vi "Calibration-Frame15.vi"(8 "Reset Measurement Prog":bool, 9 "Array 8":dbl[](array[numeric]), 10 "data mode":enum16{"Take new data point", "Refit Curve"}(ring), 11 "Results file output":path) -> ()   [LabVIEW 2022 SP3]
uses:
  Anemometry Sub Vis/Globals/Calib_global.vi
  Anemometry Sub Vis/Controls/App_Global.ctl
  Anemometry Sub Vis/Controls/Setup.ctl
  Anemometry Sub Vis/Controls/Post_Process.ctl
  Anemometry Sub Vis/Controls/Save_Data.ctl
  Anemometry Sub Vis/File/Setup_Filetype.ctl
  Anemometry Sub Vis/Globals/Meas_global.vi
  Anemometry Sub Vis/Controls/Inst_type.ctl
  Anemometry Sub Vis/Controls/portOrDev.ctl
  Anemometry Sub Vis/Controls/calType.ctl
  Anemometry Sub Vis/Controls/channelState.ctl
  Anemometry Sub Vis/Controls/Meas input Cluster.ctl
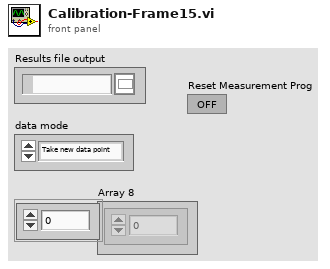
[diagram p1: front panel]
types:
  T1 = typedef "App_Global.ctl" = enum16{"Read Global", "Write to Global", "Initialise Array"}
  T2 = typedef "Save_Data.ctl" = enum16{"Save No Data", "Save Data"}
  T3 = typedef "Post_Process.ctl" = enum16{"Take New Data", "Post Process Raw Data File"}
  T4 = typedef "Setup.ctl" = enum16{"Run Program", "Show Setup", "Save Current Setup", "Setup Front Panel"}
  T5 = typedef "Setup_Filetype.ctl" = enum16{"Measurement Setups", "Calibration Setups", "General", "Results File Plotter Setups", "Speed Calib Tweaks"}
  T6 = typedef "Meas input Cluster.ctl" = cluster{"Type":T7, "Label":string, "DAQ":string, "Port":T8, "Ch":i32, "Cal":path, "calType":T9, "Fs":dbl, "syncDelay":dbl, "chState":T10}
  T7 = typedef "Inst_type.ctl" = enum16{"Raw voltage", "Raw with zero offsetting", "Propeller anemometer", "Pressure Transducer", "Pitot-static tube", "Hot wire", "Cross wire 1", "Cross wire 2", "Generic Linear", "Generic Polynomial", "Generic BackPoly", "Fast FID", "Thermocouple", "Cold wire", "Pulsed Wire", "LDA Vel", "LDA Tran time", "LDA Arr time", "Microphone"}
  T8 = typedef "portOrDev.ctl" = string
  T9 = typedef "calType.ctl" = enum32{"Latest", "Fixed"}
  T10 = typedef "channelState.ctl" = enum32{"No Selection", "Solo", "Mute"}
  T11 = typedef "Cal_Inst_type.ctl" = enum16{"Propeller anemometer", "Pressure Transducer", "Hot wire", "Cross wire velocity", "Cross wire angle", "Generic Linear", "Generic Polynomial", "Poly Fit Special", "Fast FID", "Thermocouple", "Cold wire", "Pulsed Wire"}
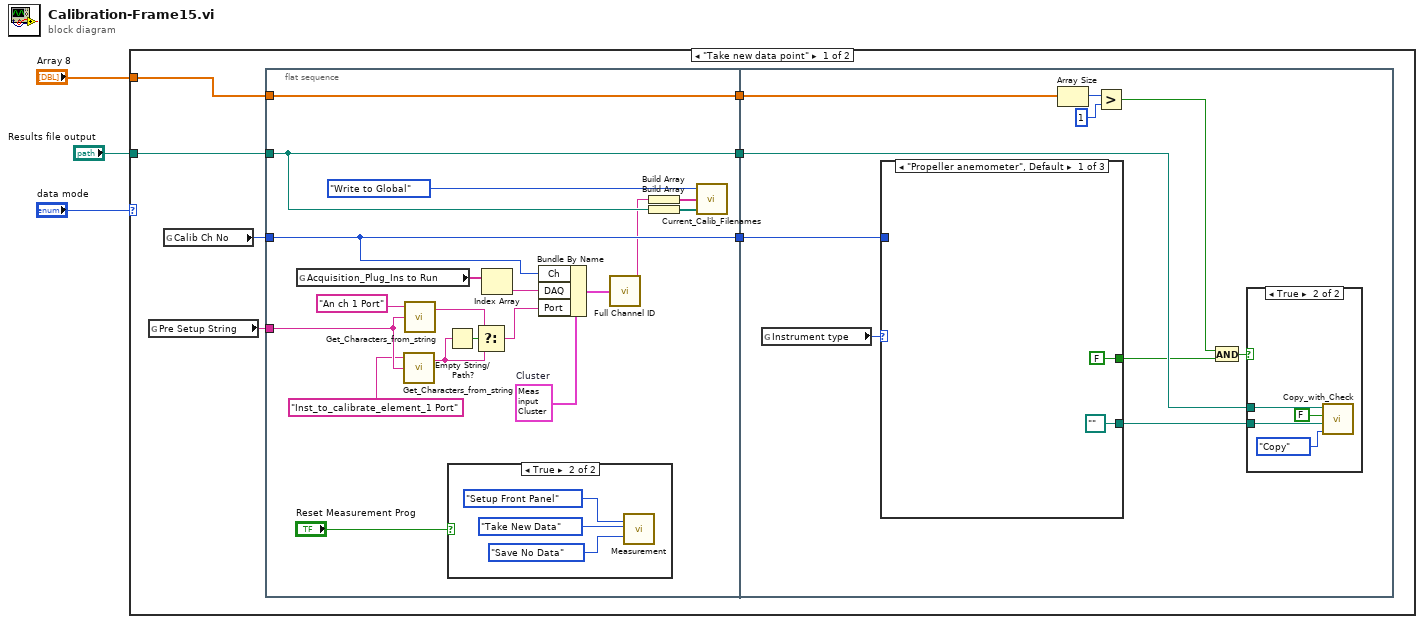
[diagram p0: block diagram]
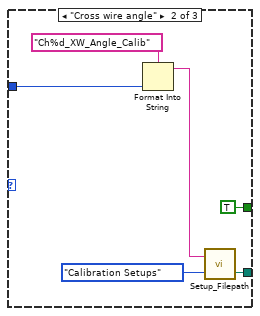
[diagram p4: hidden frame]
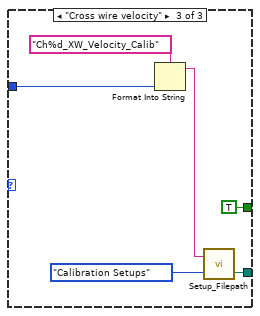
[diagram p5: hidden frame]
diagram:
  n1 = case shown="\"Take new data point\"" "data mode" {
    tunnel: "Results file output" -> [w10 _]
    tunnel: "Array 8" -> [w6 _]
    frame "Take new data point" {
      n2 = global read "Calib_global.vi" "Pre Setup String"() -> (w4:string)
      n3 = global read "Calib_global.vi" "Calib Ch No"() -> (w9:i16)
      n4 = flat-sequence {
        tunnel: w10 -> [w26]
        tunnel: [w26] -> w8
        tunnel: w9 -> [w20]
        tunnel: [w20] -> w7
        tunnel: w6 -> [w25]
        tunnel: [w25] -> w5
        tunnel: w4 -> [w17]
        tunnel: w8 -> [w40]
        tunnel: w7 -> [w34]
        tunnel: w5 -> [w33]
        frame #0 {
          w11 = T6 {"Type"=enum."Raw voltage", "Label"="", "DAQ"="", "Port"="", "Ch"=0, "Cal"=path "", "calType"=enum."Latest", "Fs"=0.0, "syncDelay"=0.0, "chState"=enum."No Selection"}  # Cluster
          n5 = global read "Meas_global.vi" "Acquisition_Plug_Ins to Run"() -> (w22:string[])
          n6 = call "Get_Characters_from_string.vi"("Input string"=w17, "Variable name"="Inst_to_calibrate_element_1 Port") -> ("Value"=w14:string)  [unwired: 1 in, 1 out]
          n7 = call "Get_Characters_from_string.vi"("Input string"=w17, "Variable name"="An ch 1 Port") -> ("Value"=w13:string)  [unwired: 1 in, 1 out]
          n8 = Empty String/Path?(string/path=w14) -> (empty?=w15:bool)
          n9 = case shown="True" "Reset Measurement Prog" {
            frame False {
            }
            frame True {
              n10 = call "Measurement.vi"("setup"=Setup."Setup Front Panel", "Post Process"=Post_Process."Take New Data", "File"=Save_Data."Save No Data") -> ()  [unwired: 3 in, 14 out]
            }
          }
          n11 = Select(t=w13, s=w15, f=w14) -> (s? t:f=w12:string)
          n12 = Index Array(array=w22) -> (element=w21:string)  [unwired: 1 in]
          n13 = Bundle By Name(cluster=w11, "Ch"=w20, "DAQ"=w21, "Port"=w12) -> (w23:T6)
          n14 = call "Full Channel ID.vi"("Cluster"=w23) -> ("String"=w19:string)
          n15 = Build Array(w19) -> (w28:string[])
          n16 = Build Array(w26) -> (w29:path[])
          n17 = call "Current_Calib_Filenames.vi"("Calib Filename"=w29, "Channel ID input"=w28, "Mode"=App_Global."Write to Global") -> ()  [unwired: 3 out]
        }
        frame #1 {
          n18 = global read "Calib_global.vi" "Instrument type"() -> (w42:T11)
          n19 = case shown="\"Propeller anemometer\", Default" w42 {
            tunnel: w34 -> [_ w54 w60]
            tunnel: [path "" ("appended path") w50 w55] -> w41
            tunnel: [FALSE TRUE TRUE] -> w37
            frame "Propeller anemometer", Default {
            }
            frame "Cross wire angle" {
              n20 = Format Into String(format string="Ch%d_XW_Angle_Calib", w54) -> (resulting string=w49:string)  [unwired: 2 in, 1 out]
              n21 = call "Setup_Filepath.vi"("Setup File Type"=Setup_Filetype."Calibration Setups", "Filename in"=w49) -> ("Filename Out"=w50:path)  [unwired: 1 out]
            }
            frame "Cross wire velocity" {
              n22 = Format Into String(format string="Ch%d_XW_Velocity_Calib", w60) -> (resulting string=w56:string)  [unwired: 2 in, 1 out]
              n23 = call "Setup_Filepath.vi"("Setup File Type"=Setup_Filetype."Calibration Setups", "Filename in"=w56) -> ("Filename Out"=w55:path)  [unwired: 1 out]
            }
          }
          n24 = Array Size(array=w33) -> (size(s)=w39:i32)
          n25 = Greater?(x=w39, y=1) -> (0:w36:bool)
          n26 = And(x=w36, y=w37) -> (x .and. y?=w35:bool)
          n27 = case shown="True" w35 {
            tunnel: w41 -> [_ w45]
            tunnel: w40 -> [_ w44]
            frame False {
            }
            frame True {
              n28 = call "Copy_with_Check.vi"("Mode"=enum16{"Move", "Copy"}."Copy", "Target Path"=w45, "Variable Target?"=FALSE, "Source Path"=w44) -> ()  [unwired: 1 out]
            }
          }
        }
      }
    }
    frame "Refit Curve" {
    }
  }
